vi "ADS1015 Read.vi"(7 "I2C Channel":u8, 8 "error in (no error)":errorcluster, 9 "ADS1015 Config Options":T1={"Channel"=4, "Expected Range (Programmable Gain Amplifier)"=0, "Sampling Mode"=1, "Sampling Rate"=4, "Comparator Mode"=1, "Comparator Polarity"=1, "Latching Comparator"=1, "Comparator Queue & Disable"=3} {"Comparator Queue & Disable" items=["Assert after one conversion", "Assert after two conversions", "Assert after four conversions", "Comparator disabled"]; "Latching Comparator" items=["Non-latching", "Latching"]; "Comparator Polarity" items=["Active Low", "Active High"]; "Comparator Mode" items=["Traditional Comparator w/ hysteresis", "Window Comparator"]; "Sampling Rate" items=["128SPS", "250SPS", "490SPS", "920SPS", "1600SPS", "2400SPS", "3300SPS"]; "Sampling Mode" items=["Continuous Conversion", "Single-shot (Low Power)"]; "Expected Range (Programmable Gain Amplifier)" items=["+/-6.144V", "+/-4.096V", "+/-2.048V", "+/-1.024V", "+/-0.512V", "+/-0.256V"]; "Channel" items=["Differential: Ch 0&1", "Differential: Ch 0&3", "Differential: Ch 1&3", "Differential: Ch 2&3", "Single Ended: Ch 0", "Single Ended: Ch 1", "Single Ended: Ch 2", "Single Ended: Ch 3"]}, 10 "I2C Slave Address":u8 format="%.0x", 11 "LINX Resource in":T2) -> (0 "error out":errorcluster, 2 "Voltage":dbl format="%.3f V", 3 "LINX Resource":T2, 4 "Resolution":dbl format="%.3f V")   [LabVIEW 2014]
uses:
  <vilib>/MakerHub/LINX/Private/Type Defs/LINX Ref.ctl
  <vilib>/MakerHub/LINX/Private/Type Defs/Platform.ctl
  <vilib>/MakerHub/LINX/Private/Type Defs/Interface.ctl
  <vilib>/MakerHub/LINX/Private/Device/Type Defs/LINX Device Config.ctl
  <vilib>/MakerHub/LINX/Private/Device/Type Defs/TCP Config.ctl
  <vilib>/MakerHub/LINX/Private/Device/Type Defs/Channels.ctl
  ADS1015 Config Options.ctl
  <vilib>/MakerHub/LINX/Private/Local IO/LinxI2cWrite.vi
  <vilib>/MakerHub/LINX/Public/Utilities/Check Channel.vi
  <vilib>/myRIO/Instrument Drivers/Onboard IO/I2C/vis/Write.vi
  <vilib>/MakerHub/LINX/Private/Utilties/Generate Error.vi
  <vilib>/MakerHub/LINX/Private/Utilties/Channel FGVs/I2C Channels.vi
  <vilib>/Utility/error.llb/Error Cluster From Error Code.vi
  <vilib>/myRIO/Common/Instrument Driver Framework/myRIO v1.0/I2C/vis/myRIO v1.0 Write I2C.vi
  <vilib>/MakerHub/LINX/LMH-LINX.lvlib
  <vilib>/MakerHub/LINX/Private/Device/Device.lvlib
panel:
  out "Raw Reading":u16 format="%.0x"
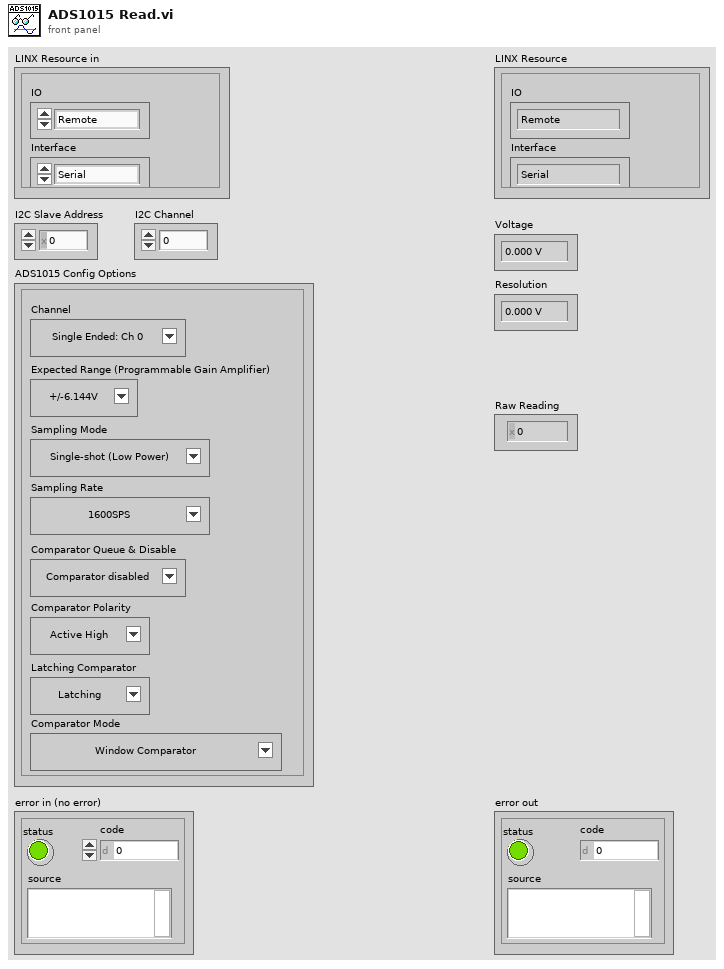
[diagram p1: front panel]
types:
  T1 = typedef "ADS1015 Config Options.ctl" = cluster{"Channel":u8, "Expected Range (Programmable Gain Amplifier)":u8, "Sampling Mode":u8, "Sampling Rate":u8, "Comparator Mode":u8, "Comparator Polarity":u8, "Latching Comparator":u8, "Comparator Queue & Disable":u8}
  T2 = typedef "LMH-LINX.lvlib/LINX Ref.ctl" = cluster{"IO":T3, "Interface":T4, "LINX Device Config":T5}
  T3 = typedef "LMH-LINX.lvlib/Platform.ctl" = enum16{"Remote", "Local"}
  T4 = typedef "LMH-LINX.lvlib/Interface.ctl" = enum16{"Serial", "TCP"}
  T5 = typedef "LMH-LINX.lvlib/Device.lvlib/LINX Device Config.ctl" = cluster{"Interface":T4, "COM Port":refnum<visa-resource-name>, "TCP Configuration":T6, "Device Family":u8, "Device ID":u8, "Device Name":string, "TCP Ref":refnum<k5>, "Channels":T7}
  T6 = typedef "LMH-LINX.lvlib/Device.lvlib/TCP Config.ctl" = cluster{"IP Address":string, "Port":u16}
  T7 = typedef "LMH-LINX.lvlib/Channels.ctl" = cluster{"DI":u8[], "DO":u8[], "AI":u8[], "AO":u8[], "PWM":u8[], "QE":u8[], "UART":u8[], "I2C 2":u8[], "SPI":u8[], "CAN":u8[], "Servo":u8[], "AI Ref (V)":dbl, "AI Resolution (Bits)":u8, "AO Ref (V)":dbl, "AO Resolution (Bits)":u8}
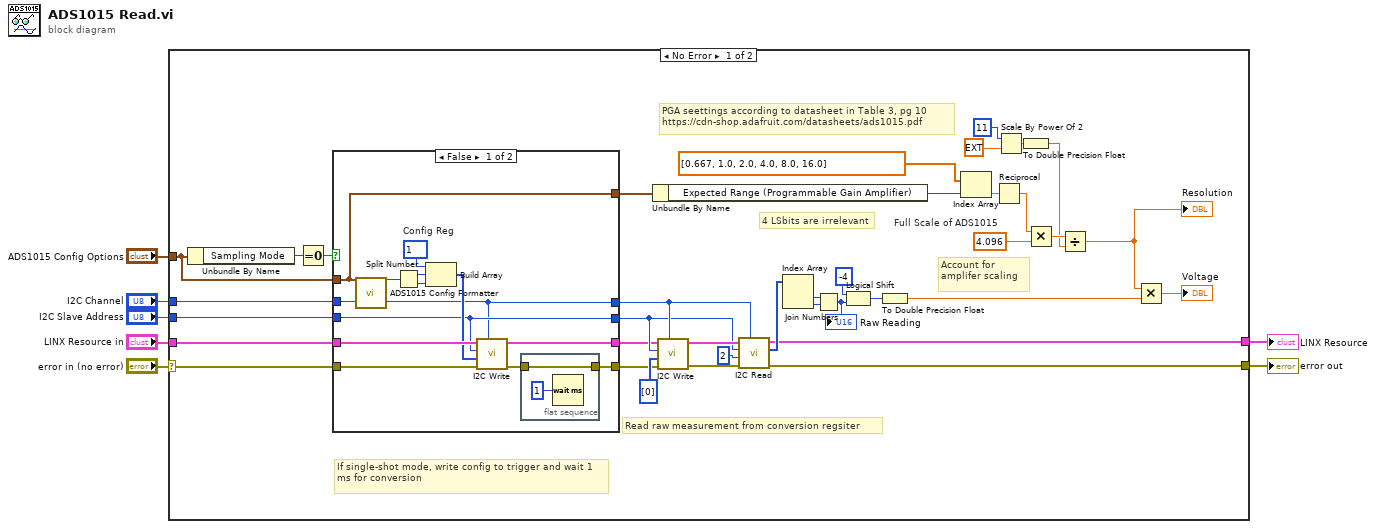
[diagram p0: block diagram]
diagram:
  n1 = case shown="No Error" "error in (no error)" {
    selector: "error in (no error)" -> [w35 w65]
    tunnel: "LINX Resource in" -> [w36 w66]
    tunnel: "I2C Channel" -> [w38 _]
    tunnel: "I2C Slave Address" -> [w37 _]
    tunnel: "ADS1015 Config Options" -> [w30 _]
    tunnel: [w28 w66] -> w2
    tunnel: [w27 w65] -> w1
    frame No Error {
      w18 = 4.096  # Full Scale of ADS1015
      # "Account for amplifer scaling"
      # "PGA seettings according to datasheet in Table 3, pg 10\nhttps://cdn-shop.adafruit.com/datasheets/ads1015.pdf"
      # "4 LSbits are irrelevant"
      # "Read raw measurement from conversion regsiter"
      # "If single-shot mode, write config to trigger and wait 1 ms for conversion"
      n2 = Unbundle By Name(w30) -> ("Sampling Mode"=w40:u8)
      n3 = Equal To 0?(x=w40) -> (x = 0?=w39:bool)
      n4 = case shown="False" w39 {
        tunnel: w38 -> [w48 w64]
        tunnel: w37 -> [w49 w63]
        tunnel: w36 -> [w53 w62]
        tunnel: w35 -> [w52 w61]
        tunnel: [w48 w64] -> w34
        tunnel: [w49 w63] -> w33
        tunnel: [w50 w62] -> w32
        tunnel: [w45 w61] -> w31
        tunnel: w30 -> [w47 w60]
        tunnel: [w47 w60] -> w23
        frame False {
          w55 = u8 1  # Config Reg
          n5 = call "ADS1015 Config Formatter.vi"("ADS1015 Config Options"=w47) -> ("Config Command"=w54:u16)  [unwired: 10 in]
          n6 = Split Number(x=w54) -> (hi(x)=w57:u8, lo(x)=w56:u8)
          n7 = Build Array(w55, w57, w56) -> (w51:u8[])
          n8 = call <vilib>:"I2C Write.vi"("I2C Channel"=w48, "Error In"=w52, "Data"=w51, "I2C Slave Address (0)"=w49, "LINX Resource"=w53) -> ("Error Out"=w46:errorcluster, "LINX Resource"=w50:T2)  [unwired: 5 in]
          n9 = flat-sequence {
            tunnel: w46 -> [w59]
            tunnel: [w59] -> w45
            frame #0 {
              n10 = Wait (ms)(milliseconds to wait=u32 1) -> ()  [unwired: 1 out]
            }
          }
        }
        frame True {
        }
      }
      n11 = Unbundle By Name(w23) -> ("Expected Range (Programmable Gain Amplifier)"=w21:u8)
      n12 = call <vilib>:"I2C Write.vi"("I2C Channel"=w34, "Error In"=w31, "Data"=u8[] [0], "I2C Slave Address (0)"=w33, "LINX Resource"=w32) -> ("Error Out"=w43:errorcluster, "LINX Resource"=w44:T2)  [unwired: 5 in]
      n13 = call <vilib>:"I2C Read.vi"("I2C Channel"=w34, "Error In"=w43, "Bytes To Read"=u8 2, "I2C Slave Address (0)"=w33, "LINX Resource"=w44) -> ("Error Out"=w27:errorcluster, "Data"=w29:u8[], "LINX Resource"=w28:T2)  [unwired: 4 in]
      n14 = Index Array(array=w29) -> (element #1=w25:u8, element #2=w26:u8)  [unwired: 2 in]
      n15 = Join Numbers(hi=w25, lo=w26) -> ((hi.lo)=w24:u16)
      "Raw Reading" <- w24
      n16 = Logical Shift(y=i16 -4, x=w24) -> (x << y=w8:u16)
      n17 = To Double Precision Float(number=w8) -> (double precision float=w16:dbl)
      n18 = Index Array(array=dbl[] [0.667, 1.0, 2.0, 4.0, 8.0, 16.0] ("Data"), index=w21) -> (element=w19:dbl)
      n19 = Reciprocal(x=w19) -> (1/x=w17:dbl)
      n20 = Scale By Power Of 2(n=i16 11, x=ext 1.0) -> (x*2^n=w11:ext)
      n21 = To Double Precision Float(number=w11) -> (double precision float=w9:dbl)
      n22 = Multiply(x=w17, y=w18) -> (x*y=w15:dbl)
      n23 = Divide(x=w15, y=w9) -> (x/y=w13:dbl)
      "Resolution" <- w13
      n24 = Multiply(x=w13, y=w16) -> (x*y=→"Voltage":dbl)
    }
    frame Error {
    }
  }
  "error out" <- w1
  "LINX Resource" <- w2
